vi "Handle Error.vi"(8 "error in (no error)":errorcluster, 11 "IMAQdx Cam Actor in":refnum<class "IMAQdx Cam Actor.lvclass">) -> (0 "error out":errorcluster, 2 "stop actor?":bool=TRUE, 3 "IMAQdx Cam Actor out":refnum<class "IMAQdx Cam Actor.lvclass">)   [LabVIEW 2014, in "IMAQdx Cam Actor.lvlib" / "IMAQdx Cam Actor.lvclass"]
doc: "(<B>Filename</B>: Actor Framework.lvlib:Actor.lvclass:Handle Error.vi)\n\nDefines how the actor handles an error that occurred while processing a message. By default, this method does nothing except stop the actor."
uses:
  IMAQdx Cam Actor.lvclass
  <vilib>/ActorFramework/Actor/Actor.lvclass
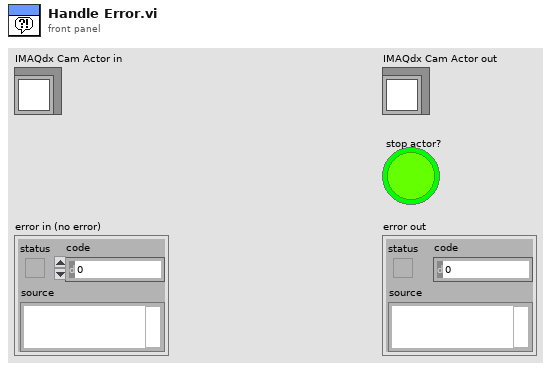
[diagram p1: front panel]
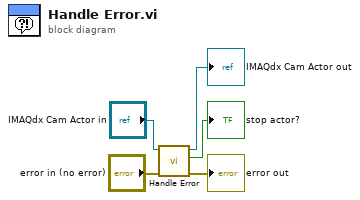
[diagram p0: block diagram]
diagram:
  n1 = call-parent "Handle Error.vi"("error in (no error)"="error in (no error)", "Actor in"="IMAQdx Cam Actor in") -> ("error out"=→"error out":errorcluster, "stop actor?"=→"stop actor?":bool, "Actor out"=→"IMAQdx Cam Actor out":refnum<class "IMAQdx Cam Actor.lvclass">)  [unwired: 7 in]
